vi "Newport ITX-D3N Assemble Data.vi"(7 "Device Number (Display In Header)":string, 8 "Error In":errorcluster, 9 "ITHX Data in":T1, 10 "iBTHX Data":T1) -> (0 "Error Out":errorcluster, 2 "Newport ITX Data":string[][](array[string]), 3 "ITHX Data out":T1)   [LabVIEW 2018]
uses:
  Type Definitions/iBTHX Data Values.ctl
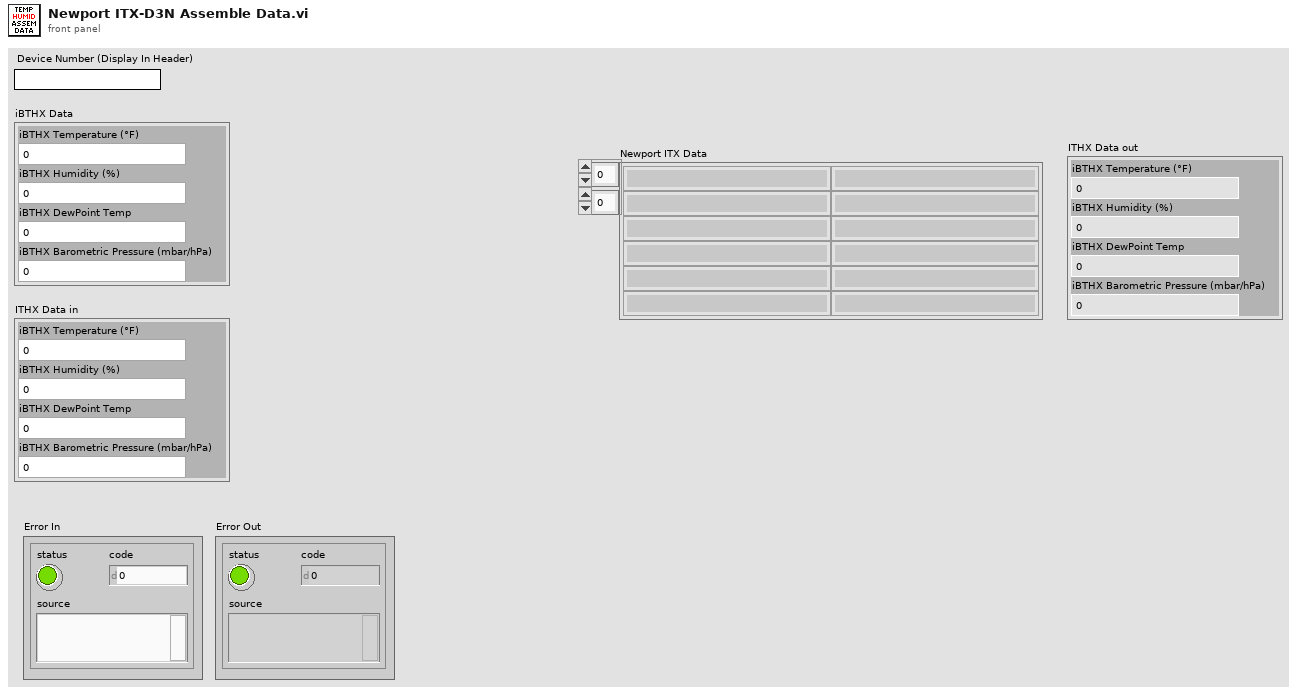
[diagram p1: front panel]
types:
  T1 = typedef "iBTHX Data Values.ctl" = cluster{"iBTHX Barometric Pressure (mbar/hPa)":dbl, "iBTHX Humidity (%)":dbl, "iBTHX Temperature (°F)":dbl, "iBTHX DewPoint Temp":dbl}
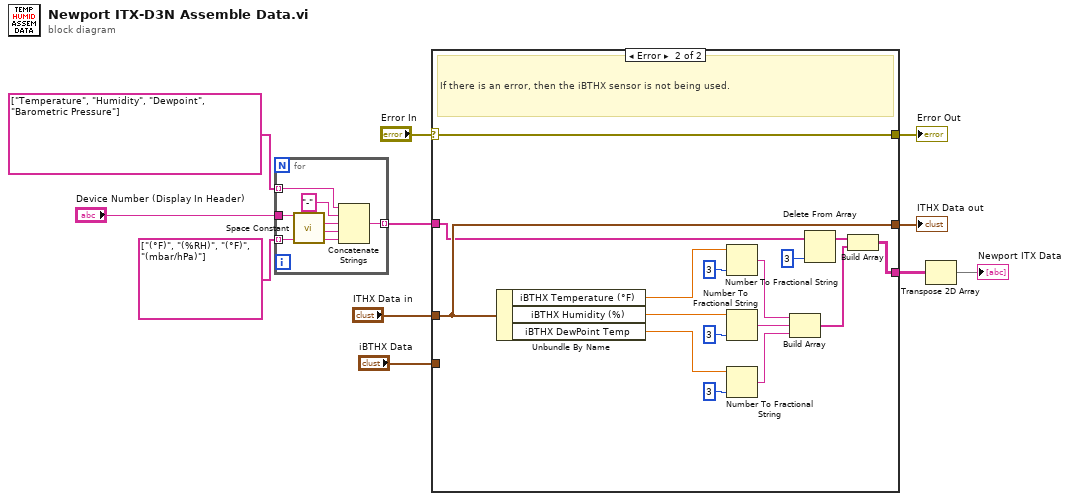
[diagram p0: block diagram]
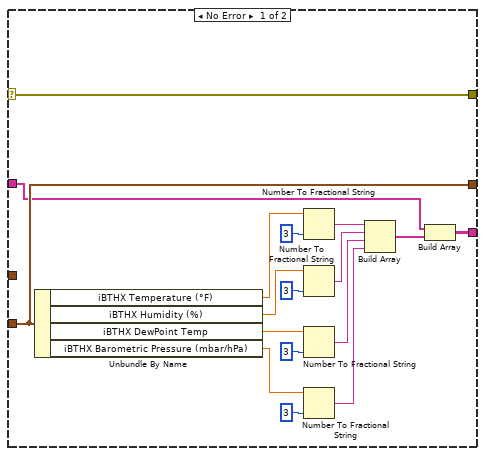
[diagram p2: hidden frame]
diagram:
  n1 = for {
    tunnel: string[] ["Temperature", "Humidity", "Dewpoint", "Barometric Pressure"] -> [w17] mode=indexing
    tunnel: "Device Number (Display In Header)" -> [w15]
    tunnel: string[] ["(°F)", "(%RH)", "(°F)", "(mbar/hPa)"] -> [w13] mode=indexing
    tunnel: [w12] -> w1 mode=indexing
    n2 = call <vilib>:"Space Constant.vi"() -> ("String"=w14:string)
    n3 = Concatenate Strings(w17, "-" ("string"), w15, w14, w13) -> (w12:string)
  }
  n4 = case shown="Error" "Error In" {
    selector: "Error In" -> [w34 w50]
    tunnel: [w34 w50] -> w6
    tunnel: "iBTHX Data" -> [w23 _]
    tunnel: [w23 w49] -> w11
    tunnel: "ITHX Data in" -> [_ w49]
    tunnel: [w19 w38] -> w8
    tunnel: w1 -> [w18 w36]
    frame No Error {
      n5 = Unbundle By Name(w23) -> ("iBTHX Temperature (°F)"=w33:dbl, "iBTHX Humidity (%)"=w29:dbl, "iBTHX DewPoint Temp"=w28:dbl, "iBTHX Barometric Pressure (mbar/hPa)"=w21:dbl)
      n6 = Number To Fractional String(number=w33, precision (6)=i16 3) -> (F-format string=w27:string)  [unwired: 2 in]
      n7 = Number To Fractional String(number=w29, precision (6)=i16 3) -> (F-format string=w26:string)  [unwired: 2 in]
      n8 = Number To Fractional String(number=w28, precision (6)=i16 3) -> (F-format string=w25:string)  [unwired: 2 in]
      n9 = Number To Fractional String(number=w21, precision (6)=i16 3) -> (F-format string=w20:string)  [unwired: 2 in]
      n10 = Build Array(w27, w26, w25, w20) -> (w24:string[])
      n11 = Build Array(w18, w24) -> (w19:string[][])
    }
    frame Error {
      # "If there is an error, then the iBTHX sensor is not being used."
      n12 = Unbundle By Name(w49) -> ("iBTHX Temperature (°F)"=w48:dbl, "iBTHX Humidity (%)"=w44:dbl, "iBTHX DewPoint Temp"=w43:dbl)
      n13 = Number To Fractional String(number=w48, precision (6)=i16 3) -> (F-format string=w42:string)  [unwired: 2 in]
      n14 = Number To Fractional String(number=w44, precision (6)=i16 3) -> (F-format string=w41:string)  [unwired: 2 in]
      n15 = Number To Fractional String(number=w43, precision (6)=i16 3) -> (F-format string=w40:string)  [unwired: 2 in]
      n16 = Build Array(w42, w41, w40) -> (w39:string[])
      n17 = Delete From Array(array=w36, index=3) -> (array with subset deleted=w35:string[])  [unwired: 1 in, 1 out]
      n18 = Build Array(w35, w39) -> (w38:string[][])
    }
  }
  "ITHX Data out" <- w11
  "Error Out" <- w6
  n19 = Transpose 2D Array(2D array=w8) -> (transposed array=→"Newport ITX Data":string[][])
